vi "PIDApplication.vi"() -> ()   [LabVIEW 2019]
uses:
  <vilib>/Platform/TimedLoop/XDataNode/timing_clust.ctl
  <vilib>/Platform/TimedLoop/XDataNode/nitl_modes.ctl
  <vilib>/Platform/TimedLoop/XDataNode/wakeup.ctl
  <vilib>/Instr/_visa.llb/VISA Configure Serial Port (Instr).vi
  GblVariableForLogging.vi
  <vilib>/Utility/file.llb/Write Delimited Spreadsheet (DBL).vi
  <vilib>/platform/TimedLoop/XDataNode/XDataNode.xnode
  <vilib>/Platform/TimedLoop/XDataNode/XDNodeRunTimeDep.lvlib
panel:
  out "Waveform Chart":T1(graph)
  in  "stop":bool
  in  "VISA resource name":refnum<visa-resource-name>="COM1"
  in  "Set point":u8
  in  "Freq":u8
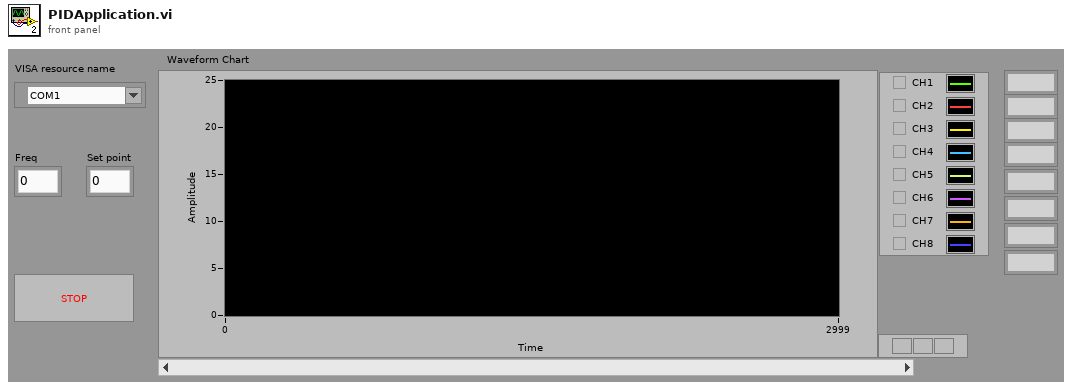
[diagram p1: front panel]
types:
  T1 = cluster{"TempOutput":dbl, "TempOutput":dbl, "TempOutput":dbl, "TempOutput":dbl, "TempOutput":dbl, "TempOutput":dbl, "TempOutput":dbl, "TempOutput":dbl}
  T2 = cluster{"Output":u16, "Output":u16, "Output":u16, "Output":u16, "Output":u16, "Output":u16, "Output":u16, "Output":u16}[]
  T3 = typedef "XDNodeRunTimeDep.lvlib/timing_clust.ctl" = cluster{"Expected End [f-1]":u64, "Actual End [f-1]":u64, "Finished Late? [f-1]":bool, "Expected End [i-1]":u64, "Actual End [i-1]":u64, "Finished Late? [i-1]":bool, "Expected Start [i]":u64, "Actual Start [i]":u64, "Expected Start [f]":u64, "Actual Start [f]":u64, "Source Name":string, "Structure Name":string, "Period":i64, "Deadline":i64, "Offset":i64, "Start":i64, "Priority":i32, "Timeout":i32, "Mode":T4, "Wakeup Reason":T5, "Error":errorcluster, "Source Type":string, "Secondary Source Type":string, "Global End Time":u64, "Global Start Time":u64, "Frame Duration":u64, "Iteration Duration":u64, "Assigned CPU":i32, "I/O Scan Engine Mode":u32}
  T4 = typedef "XDNodeRunTimeDep.lvlib/nitl_modes.ctl" = enum32{"No Change", "Process missed periods, maintain original phase", "Discard missed periods, maintain original phase", "Process missed periods, ignore original phase", "Discard missed periods, ignore original phase"}
  T5 = typedef "XDNodeRunTimeDep.lvlib/wakeup.ctl" = enum32{"Normal", "Aborted", "Asynchronous wakeup", "Timing source error", "Timed loop error", "Timeout"}
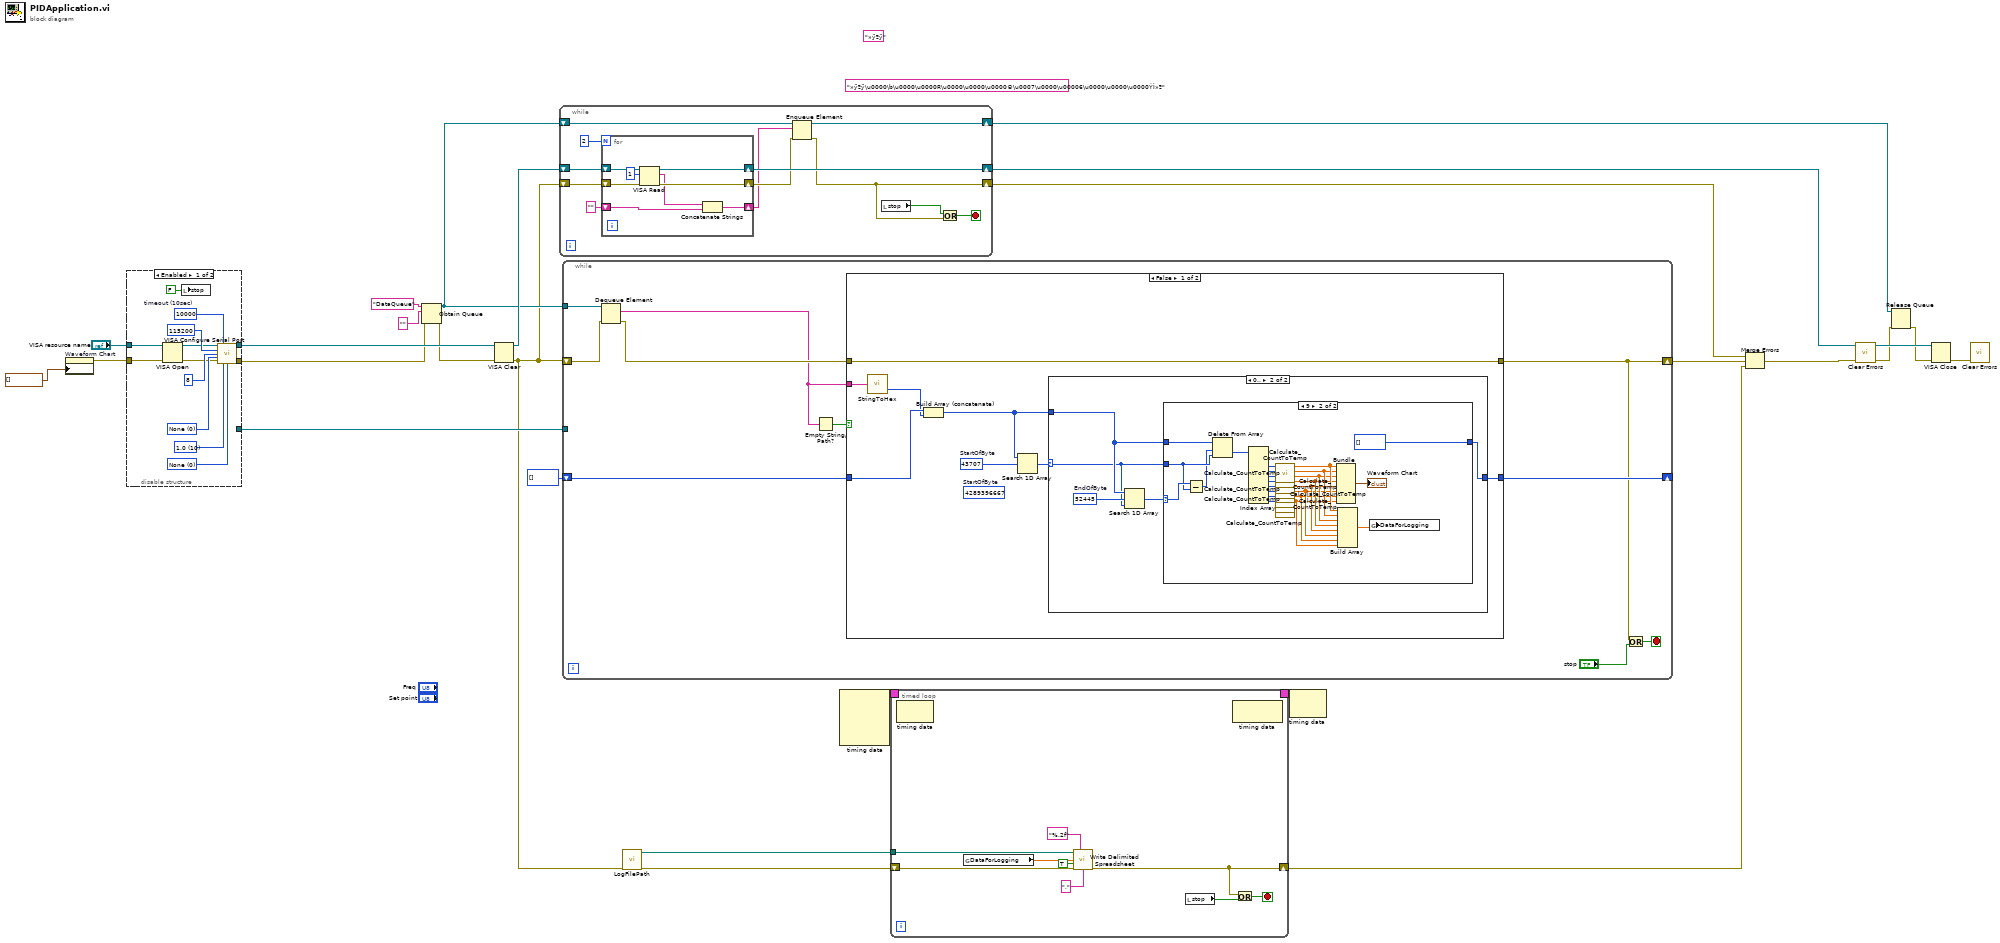
[diagram p0: block diagram]
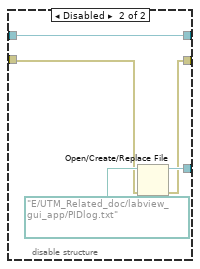
[diagram p2: hidden frame]
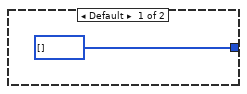
[diagram p3: hidden frame]
diagram:
  (unwired) "»ÿªÿ"
  (unwired) "»ÿªÿ\u0000\b\u0000\u0000R\u0000\u0000\u0000®\u0007\u0000\u00006\u0000\u0000\u0000ÝÌ»ª"
  n1 = property on="Waveform Chart" class="WFChart (strict)"("History Data"=T2 []) -> (error out=w24:errorcluster)  [unwired: 2 in, 1 out]
  n2 = disable-structure shown="Enabled" {
    disable-tunnel: "VISA resource name" -> [w33 w44]
    disable-tunnel: [w30 w44] -> w21
    disable-tunnel: [w29 w40] -> w7
    disable-tunnel: w24 -> [w28 w41]
    disable-tunnel: [_ w42] -> w23
    frame Enabled {
      w35 = u16 0 items=["None"=0, "XON/XOFF"=1, "RTS/CTS"=2, "DTR/DSR"=4] ("flow control")
      w36 = u16 10 items=["1.0"=10, "1.5"=15, "2.0"=20] ("stop bits")
      w38 = u16 0 items=["None", "Odd", "Even", "Mark", "Space"] ("parity")
      w37 = u32 10000  # timeout (10sec)
      n3 = VISA Open(error in (no error)=w28, VISA resource name=w33) -> (VISA resource name=w32:refnum<visa-resource-name>, error out=w31:errorcluster)  [unwired: 3 in]
      n4 = local write "stop"(FALSE ("stop")) -> ()
      n5 = call-poly "VISA Configure Serial Port"("VISA resource name"=w32, "timeout (10sec)"=w37, "baud rate (9600)"=u32 115200 ("baud rate"), "data bits (8)"=u16 8 ("data bits"), "parity (0:none)"=w38, "error in (no error)"=w31, "stop bits (10: 1 bit)"=w36, "flow control (0:none)"=w35) -> ("VISA resource name out"=w30:refnum<visa-resource-name>, "error out"=w29:errorcluster)  [unwired: 1 in, 5 out]
    }
    frame Disabled {
      n6 = Open/Create/Replace File(file path (use dialog)=path "E:/UTM_Related_doc/labview_gui_app/PIDlog.txt", error in=w41) -> (refnum out=w42:refnum<file>, error out=w40:errorcluster)  [unwired: 4 in, 1 out]
    }
  }
  n7 = Obtain Queue(name (unnamed)="DataQueue", element data type="", error in (no error)=w7) -> (queue out=w13:refnum<queue>, error out=w14:errorcluster)  [unwired: 2 in, 1 out]
  n8 = VISA Clear(VISA resource name=w21, error in (no error)=w14) -> (VISA resource name out=w20:refnum<visa-resource-name>, error out=w3:errorcluster)
  n9 = while {
    shift-right: [w51] -> w19
    shift-left: w20 -> [w50]
    shift-right: [w47] -> w18
    shift-left: w3 -> [w55]
    shift-right: [w45] -> w9
    shift-left: w13 -> [w49]
    stop <- w52 stop-if-true
    n10 = for {
      N: 2 -> [_]
      shift-right: [w62] -> w51
      shift-left: w50 -> [w64]
      shift-right: [w63] -> w48
      shift-left: w55 -> [w61]
      shift-right: [w59] -> w46
      shift-left: "" -> [w57]
      n11 = VISA Read(VISA resource name=w64, byte count=u32 1, error in (no error)=w61) -> (VISA resource name out=w62:refnum<visa-resource-name>, read buffer=w58:string, error out=w63:errorcluster)  [unwired: 1 out]
      n12 = Concatenate Strings(w58, w57) -> (w59:string)
    }
    n13 = Enqueue Element(queue=w49, element=w46, error in (no error)=w48) -> (queue out=w45:refnum<queue>, error out=w47:errorcluster)  [unwired: 1 in, 1 out]
    n14 = local read "stop"() -> (w53:bool)
    n15 = Or(x=w53, y=w47) -> (x .or. y?=w52:bool)
  }
  n16 = while {
    shift-right: [w72] -> w17
    shift-left: w3 -> [w67]
    shift-right: [w73] -> _
    shift-left: u16[] [] ("OutputDecimal") -> [w74]
    tunnel: w23 -> [_]
    tunnel: w13 -> [w68]
    stop <- w71 stop-if-true
    n17 = Dequeue Element(queue=w68, error in (no error)=w67) -> (element=w65:string, error out=w66:errorcluster)  [unwired: 1 in, 2 out]
    n18 = Empty String/Path?(string/path=w65) -> (empty?=w69:bool)
    n19 = case shown="False" w69 {
      tunnel: [w78 w115] -> w72
      tunnel: w66 -> [w78 w115]
      tunnel: [w80 w114] -> w73
      tunnel: w74 -> [w79 w114]
      tunnel: w65 -> [w77 _]
      frame False {
        (unwired) u32 4289396667  # StartOfByte
        w82 = u16 43707  # StartOfByte
        n20 = call "StringToHex.vi"("Input String"=w77) -> ("Output"=w75:u16)  [unwired: 1 out]
        n21 = Build Array (concatenate)(w79, w75) -> (w76:u16[])
        n22 = Search 1D Array(1D array=w76, element=w82) -> (index of element=w81:i32)  [unwired: 1 in]
        n23 = case shown="0.." w81 {
          selector: w81 -> [_ w85]
          tunnel: [u16[] [] w84] -> w80
          tunnel: w76 -> [_ w86]
          frame Default {
          }
          frame 0.. {
            w88 = u16 52445  # EndOfByte
            n24 = Search 1D Array(1D array=w86, element=w88, start index (0)=w85) -> (index of element=w87:i32)
            n25 = case shown="9" w87 {
              selector: w87 -> [_ w112]
              tunnel: w86 -> [w89 w113]
              tunnel: w85 -> [_ w111]
              tunnel: [w89 u16[] []] -> w84
              frame Default {
              }
              frame 9 {
                n26 = Subtract(x=w112, y=w111) -> (x-y=w110:i32)
                n27 = Delete From Array(array=w113, length=w110, index=w111) -> (deleted portion=w99:u16[])  [unwired: 1 out]
                n28 = Index Array(array=w99) -> (element #2=w107:u16, element #3=w106:u16, element #4=w105:u16, element #5=w104:u16, element #6=w103:u16, element #7=w102:u16, element #8=w101:u16, element #9=w100:u16)  [unwired: 9 in, 1 out]
                n29 = call "Calculate_CountToTemp.vi"("CountInput"=w107) -> ("TempOutput"=w98:dbl)  [unwired: 10 in]
                n30 = call "Calculate_CountToTemp.vi"("CountInput"=w106) -> ("TempOutput"=w96:dbl)  [unwired: 10 in]
                n31 = call "Calculate_CountToTemp.vi"("CountInput"=w105) -> ("TempOutput"=w95:dbl)  [unwired: 10 in]
                n32 = call "Calculate_CountToTemp.vi"("CountInput"=w104) -> ("TempOutput"=w94:dbl)  [unwired: 10 in]
                n33 = call "Calculate_CountToTemp.vi"("CountInput"=w103) -> ("TempOutput"=w93:dbl)  [unwired: 10 in]
                n34 = call "Calculate_CountToTemp.vi"("CountInput"=w102) -> ("TempOutput"=w92:dbl)  [unwired: 10 in]
                n35 = call "Calculate_CountToTemp.vi"("CountInput"=w101) -> ("TempOutput"=w91:dbl)  [unwired: 10 in]
                n36 = call "Calculate_CountToTemp.vi"("CountInput"=w100) -> ("TempOutput"=w90:dbl)  [unwired: 10 in]
                n37 = Bundle("TempOutput"=w98, "TempOutput"=w96, "TempOutput"=w95, "TempOutput"=w94, "TempOutput"=w93, "TempOutput"=w92, "TempOutput"=w91, "TempOutput"=w90) -> (→"Waveform Chart":T1)  [unwired: 1 in]
                n38 = Build Array(w98, w96, w95, w94, w93, w92, w91, w90) -> (w97:dbl[])
                n39 = global write "GblVariableForLogging.vi" "DataForLogging"(w97) -> ()
              }
            }
          }
        }
      }
      frame True {
      }
    }
    n40 = Or(x=w72, y="stop") -> (x .or. y?=w71:bool)
  }
  n41 = call "LogFilePath.vi"("error in (no error)"=w3) -> ("error out"=w2:errorcluster, "appended path"=w1:path)  [unwired: 9 in]
  n42 = node-c288() -> (w5:T3)  [unwired: 4 in]
  n43 = timed-loop {
    shift-right: [w122] -> w6
    shift-left: w2 -> [w121]
    timing: w5 -> [_]
    timing-out: [_] -> w4
    tunnel: w1 -> [w117]
    stop <- w123 stop-if-true
    n44 = node-c288() -> ()  [unwired: 1 in, 1 out]
    n45 = global read "GblVariableForLogging.vi" "DataForLogging"() -> (w120:dbl[])
    n46 = call-poly <vilib>:"Write Delimited Spreadsheet.vi"("file path (dialog if empty)"=w117, "format (%.3f)"="%.2f", "1D data"=w120, "append to file? (new file:F)"=TRUE, "error in (no error)"=w121, "delimiter (\\t)"="," ("delimiter (\\t)")) -> ("error out"=w122:errorcluster)  [unwired: 8 in, 1 out]
    n47 = local read "stop"() -> (w124:bool)
    n48 = node-c288() -> ()  [unwired: 1 in, 1 out]
    n49 = Or(x=w122, y=w124) -> (x .or. y?=w123:bool)
  }
  n50 = node-c288(w4) -> ()  [unwired: 1 out]
  n51 = Merge Errors(w18, w17, w6) -> (w16:errorcluster)
  n52 = call <vilib>:"Clear Errors.vi"("error in (no error)"=w16) -> ("error out"=w11:errorcluster)  [unwired: 5 in, 1 out]
  n53 = Release Queue(queue=w9, error in (no error)=w11) -> (error out=w10:errorcluster)  [unwired: 1 in, 2 out]
  n54 = VISA Close(VISA resource name=w19, error in (no error)=w10) -> (error out=w25:errorcluster)
  n55 = call <vilib>:"Clear Errors.vi"("error in (no error)"=w25) -> ()  [unwired: 5 in, 2 out]
